vi "AssertIndexValue.vi"(0 "VI Reference In":refnum<vi>, 1 "Test Label":string, 2 "delimiter (>>)":string=">>", 3 "Assert Only? (F)":bool, 5 "Control Path":string, 7 "Item Index":i32, 9 "Item Value":string, 11 "Error In":errorcluster, 12 "Assert Interval(10 ms)":u32=10, 13 "Timeout(5 sec)":dbl=5.0) -> (4 "VI Reference Out":refnum<vi>, 6 "Asserted Value":string, 15 "Error Out":errorcluster)   [LabVIEW 2016, in "Drona.lvlib" / "AssertControlValue.lvlib" / "AssertListbox.lvlib"]
doc: "Asserts if the item name on specified index in the listbox control is equal.\n\nThe input control name is given as a string , incase of path, use delimiters inbetween the path.\nThis VI gets the value of the control, untill the value is equal to the input value."
uses:
  AssertListbox.lvlib
  Get/GetControlRef/GetControlRefByPath.vi
  <vilib>/Utility/error.llb/Error Cluster From Error Code.vi
  <vilib>/addons/_JKI Toolkits/Caraya/classes/Assert/Assert Equal Value_Variant.vi
  <vilib>/ErrorRing/Error Ring.xnode
  <vilib>/addons/_JKI Toolkits/Caraya/classes/Assert/Assert.lvclass
  Get/GetControlRef/GetControlRef.lvlib
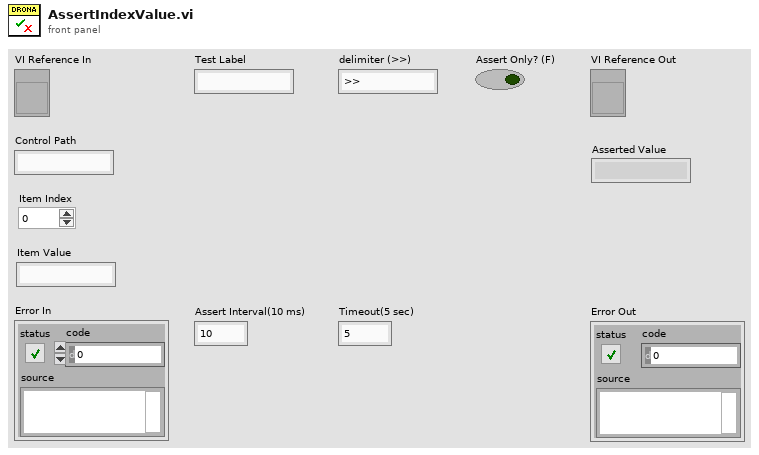
[diagram p1: front panel]
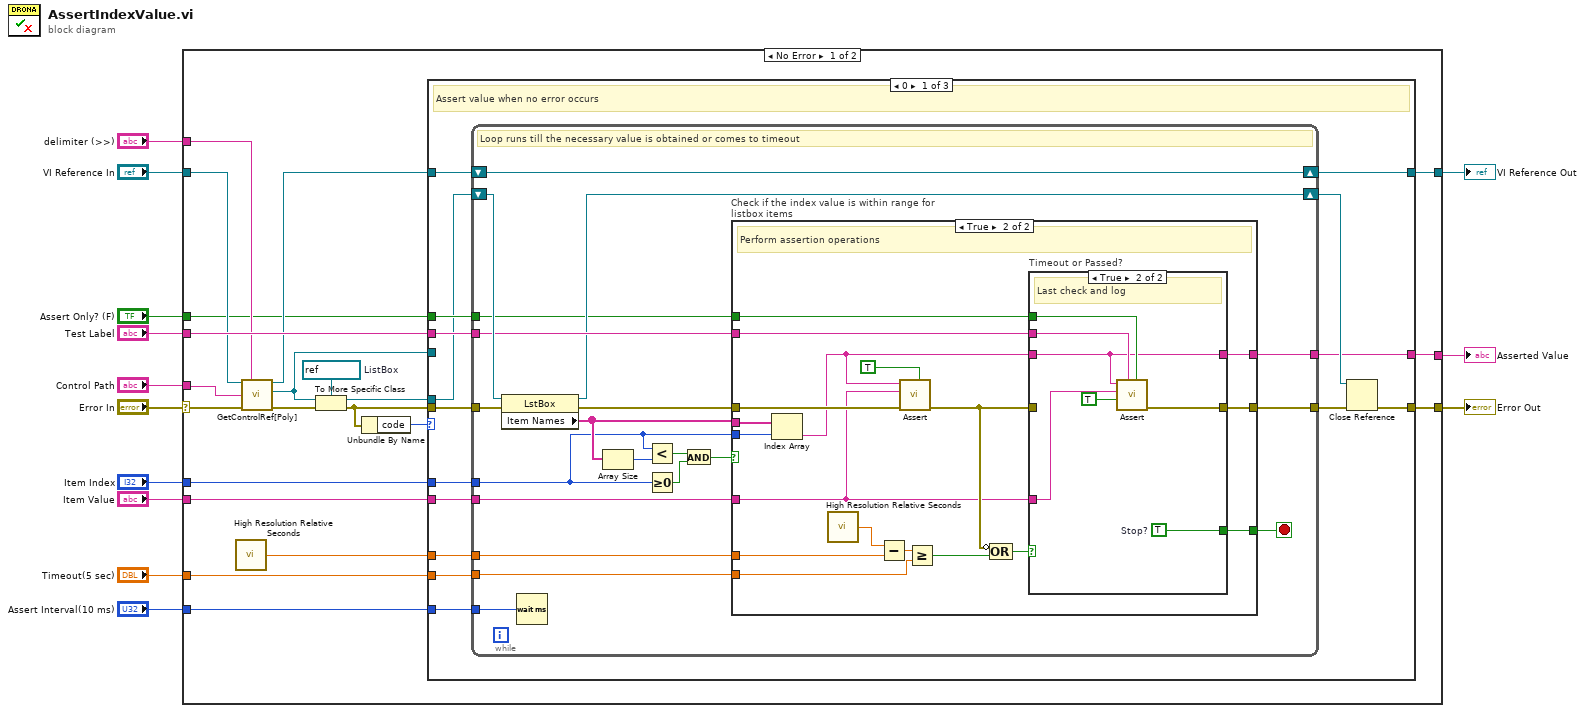
[diagram p0: block diagram]
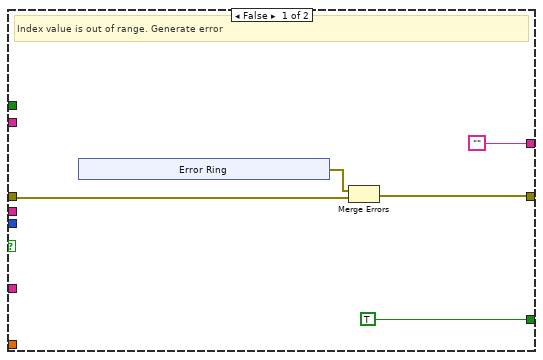
[diagram p2: hidden frame]
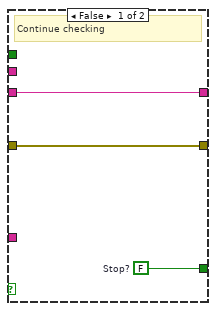
[diagram p3: hidden frame]
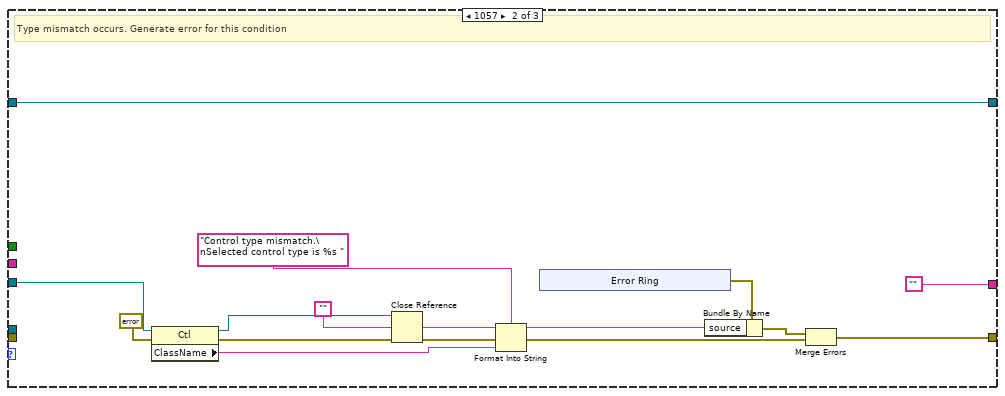
[diagram p4: hidden frame]
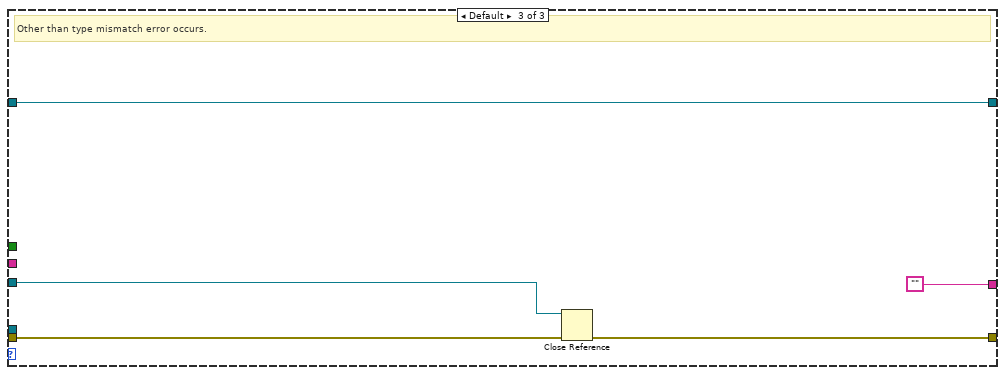
[diagram p5: hidden frame]
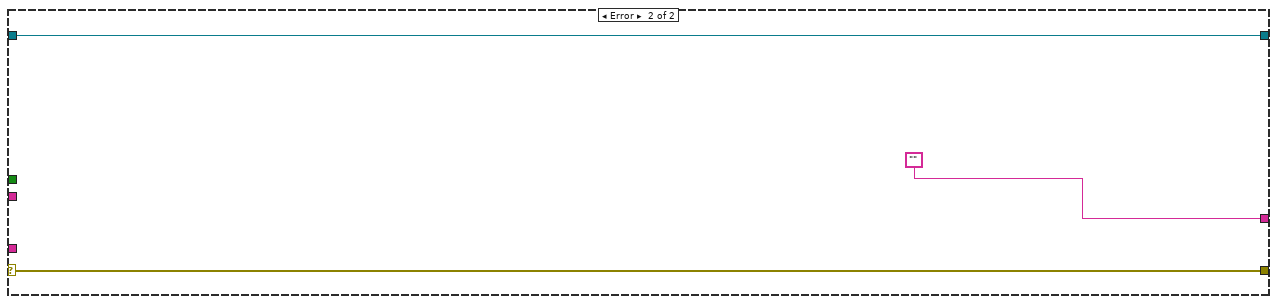
[diagram p6: hidden frame]
diagram:
  n1 = case shown="No Error" "Error In" {
    selector: "Error In" -> [w29 w135]
    tunnel: "Timeout(5 sec)" -> [w34 _]
    tunnel: [w33 w134] -> w12
    tunnel: "Item Index" -> [w32 _]
    tunnel: [w23 w135] -> w11
    tunnel: "Assert Interval(10 ms)" -> [w31 _]
    tunnel: "Test Label" -> [w30 _]
    tunnel: "VI Reference In" -> [w28 w134]
    tunnel: "Control Path" -> [w27 _]
    tunnel: "delimiter (>>)" -> [w22 _]
    tunnel: "Assert Only? (F)" -> [w21 _]
    tunnel: [w20 ""] -> w1
    tunnel: "Item Value" -> [w17 _]
    frame No Error {
      w19 = refnum<vi> refnum  # ListBox
      n2 = call <vilib>:"High Resolution Relative Seconds.vi"() -> ("relative seconds"=w26:dbl)
      n3 = call-poly "GetControlRef[Poly].vi"("VI Reference In"=w28, "delimiter (>>)"=w22, "Control Path"=w27, "error In"=w29) -> ("VI Reference Out"=w24:refnum<vi>, "Ctl Refnum"=w14:refnum<vi>, "error out"=w25:errorcluster)  [unwired: 9 in]
      n4 = To More Specific Class(target class=w19, reference=w14, error in=w25) -> (specific class reference=w18:refnum<vi>, error out=w16:errorcluster)
      n5 = Unbundle By Name(w16) -> ("code"=w15:i32)
      n6 = case shown="0" w15 {
        tunnel: w34 -> [w49 _ _]
        tunnel: [w48 w121 w132] -> w33
        tunnel: w32 -> [w47 _ _]
        tunnel: w31 -> [w45 _ _]
        tunnel: w30 -> [w44 _ _]
        tunnel: w26 -> [w43 _ _]
        tunnel: w24 -> [w42 w121 w132]
        tunnel: [w41 w109 w129] -> w23
        tunnel: w21 -> [w39 _ _]
        tunnel: [w38 "" ""] -> w20
        tunnel: w16 -> [w37 _ w131]
        tunnel: w18 -> [w36 _ _]
        tunnel: w17 -> [w35 _ _]
        tunnel: w14 -> [_ w108 w128]
        frame 0 {
          # "Assert value when no error occurs"
          n7 = while {
            tunnel: w47 -> [w53]
            tunnel: w49 -> [w68]
            tunnel: w43 -> [w69]
            tunnel: w37 -> [w63]
            tunnel: [w66] -> w46
            tunnel: w45 -> [w64]
            tunnel: w44 -> [w60]
            shift-right: [w61] -> w48
            shift-left: w42 -> [w61]
            shift-right: [w59] -> w40
            shift-left: w36 -> [w62]
            tunnel: w39 -> [w58]
            tunnel: [w57] -> w38
            tunnel: w35 -> [w56]
            stop <- w67 stop-if-true
            # "Loop runs till the necessary value is obtained or comes to timeout"
            n8 = property on="Property Node" class="LstBox"(reference=w62, error in=w63) -> (reference out=w59:refnum<vi>, error out=w65:errorcluster, "Item Names"=w55:string[])
            n9 = Wait (ms)(milliseconds to wait=w64) -> ()  [unwired: 1 out]
            n10 = Array Size(array=w55) -> (size(s)=w54:i32)
            n11 = Less?(x=w53, y=w54) -> (x < y?=w51:bool)
            n12 = Greater Or Equal To 0?(x=w53) -> (x >= 0?=w52:bool)
            n13 = And(x=w51, y=w52) -> (x .and. y?=w50:bool)
            n14 = case "Check if the index value is within range for listbox items" shown="True" w50 {
              tunnel: w69 -> [_ w97]
              tunnel: w68 -> [_ w94]
              tunnel: [TRUE w86] -> w67
              tunnel: [w70 w87] -> w66
              tunnel: w60 -> [_ w92]
              tunnel: w58 -> [_ w85]
              tunnel: ["" w84] -> w57
              tunnel: w56 -> [_ w83]
              tunnel: w55 -> [_ w82]
              tunnel: w53 -> [_ w80]
              tunnel: w65 -> [w71 w93]
              frame False {
                # "Index value is out of range. Generate error"
                n15 = xnode "Error Ring"() -> ("error out"=w72:errorcluster)
                n16 = Merge Errors(w72, w71) -> (w70:errorcluster)
              }
              frame True {
                # "Perform assertion operations"
                n17 = Index Array(array=w82, index=w80) -> (element=w81:string)
                n18 = call <vilib>:"High Resolution Relative Seconds.vi"() -> ("relative seconds"=w96:dbl)
                n19 = Subtract(x=w96, y=w97) -> (x-y=w95:dbl)
                n20 = call-poly <vilib>:"Assert.vi"("Assert Only? (F)"=TRUE, "error in (no error)"=w93, "Y"=w83, "X"=w81) -> ("error out"=w90:errorcluster)  [unwired: 7 in]
                n21 = Greater Or Equal?(x=w95, y=w94) -> (x >= y?=w91:bool)
                n22 = Compound Arithmetic op=OR(invert w90, w91) -> (w89:bool)
                n23 = case "Timeout or Passed?" shown="True" w89 {
                  tunnel: w90 -> [w100 _]
                  tunnel: w83 -> [_ w106]
                  tunnel: w81 -> [w98 w101]
                  tunnel: w92 -> [_ w107]
                  tunnel: [w100 w105] -> w87
                  tunnel: [w99 w104] -> w86
                  tunnel: w85 -> [_ w102]
                  tunnel: [w98 w101] -> w84
                  frame False {
                    w99 = FALSE  # Stop?
                    # "Continue checking"
                  }
                  frame True {
                    w104 = TRUE  # Stop?
                    # "Last check and log"
                    n24 = call-poly <vilib>:"Assert.vi"("Assert Only? (F)"=w102, "Label"=w107, "Register with caller test (F)"=TRUE, "Y"=w106, "X"=w101) -> ("error out"=w105:errorcluster)  [unwired: 6 in]
                  }
                }
              }
            }
          }
          n25 = Close Reference(reference=w40, error in (no error)=w46) -> (error out=w41:errorcluster)
        }
        frame 1057 {
          # "Type mismatch occurs. Generate error for this condition"
          n26 = property class="Ctl"(reference=w108, error in=errorcluster {"status"=FALSE, "code"=0, "source"=""} ("error out")) -> (reference out=w110:refnum<vi>, error out=w120:errorcluster, "ClassName"=w117:string)
          n27 = Close Reference(reference=w110, error in (no error)=w120) -> (error out=w111:errorcluster)
          n28 = Format Into String(format string="Control type mismatch.\nSelected control type is %s ", initial string="", error in=w111, w117) -> (resulting string=w114:string, error out=w112:errorcluster)
          n29 = xnode "Error Ring"() -> ("error out"=w115:errorcluster)
          n30 = Bundle By Name(cluster=w115, "source"=w114) -> (w113:errorcluster)
          n31 = Merge Errors(w113, w112) -> (w109:errorcluster)
        }
        frame Default {
          # "Other than type mismatch error occurs."
          n32 = Close Reference(reference=w128, error in (no error)=w131) -> (error out=w129:errorcluster)
        }
      }
    }
    frame Error {
    }
  }
  "Error Out" <- w11
  "VI Reference Out" <- w12
  "Asserted Value" <- w1
